vi "GetType.vi"(8 "error in (no error)":errorcluster, 11 "Start Pattern Msg":refnum<class "Start Pattern Msg.lvclass">) -> (0 "error out":errorcluster, 2 "Data Sample":variant, 3 "Start Pattern Msg":refnum<class "Start Pattern Msg.lvclass">)   [LabVIEW 2015, in "CS++PPG.lvlib" / "Start Pattern Msg.lvclass"]
uses:
  Start Pattern Msg.lvclass
  Start Pattern Msg.lvclass/Start Pattern Msg.ctl
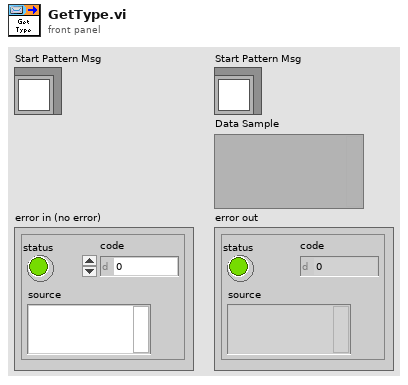
[diagram p1: front panel]
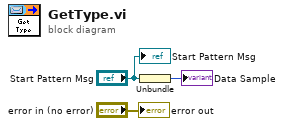
[diagram p0: block diagram]
diagram:
  n1 = Unbundle("Start Pattern Msg") -> (→"Data Sample":i32)
  "error out" <- "error in (no error)"
  "Start Pattern Msg" <- "Start Pattern Msg"
